vi "Event Messenger Priority_DialogHelp.vi"() -> ()   [LabVIEW 2020]
panel:
  out "String 2":string="Event Messenger Priority : a channel that allows each Write operation to trigger an event in Event Structures.\nA message holds it's priority it was send with."
  out "Context Help":string
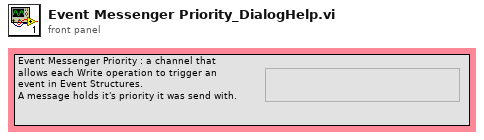
[diagram p1: front panel]
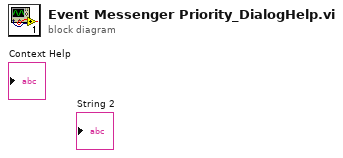
[diagram p0: block diagram]
diagram:
